vi "Picolog Get Unit Info.vi"(8 "Error In":errorcluster, 11 "Instrument Handle In":i16=1) -> (0 "Error Out":errorcluster, 1 "Unit Info":string, 3 "Instrument Handle Out":i16)   [LabVIEW 2016]
uses:
  usbtc08.dll
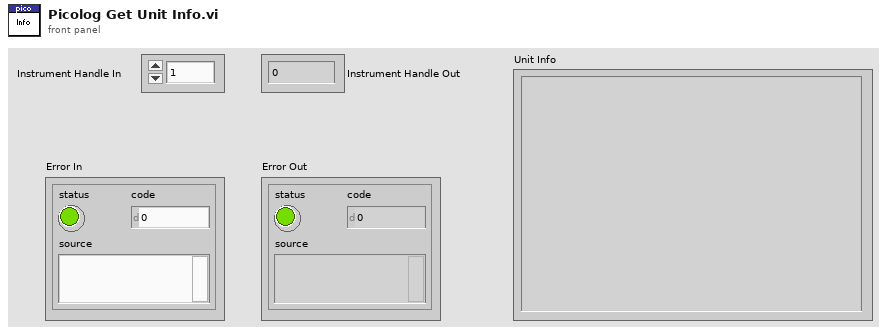
[diagram p1: front panel]
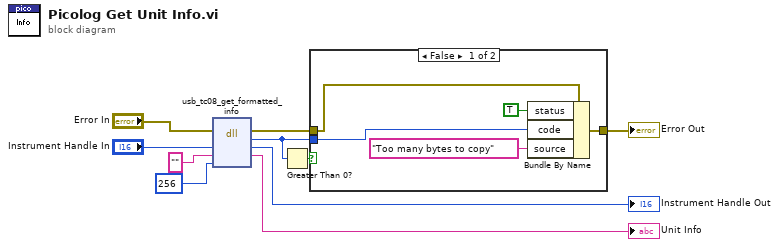
[diagram p0: block diagram]
diagram:
  n1 = dll-call lib="usbtc08.dll" fn="usb_tc08_get_formatted_info"(error in="Error In", "handle"="Instrument Handle In", "info"="", "string_length"=i16 256 ("String Length")) -> (error out=w7:errorcluster, "return type"=w3:i16, "handle"=→"Instrument Handle Out":i16, "info"=→"Unit Info":string)  [unwired: 3 in, 1 out]
  n2 = Greater Than 0?(x=w3) -> (x > 0?=w8:bool)
  n3 = case shown="False" w8 {
    tunnel: w7 -> [w15 w16]
    tunnel: [w14 w16] -> w6
    tunnel: w3 -> [w11 _]
    frame False {
      n4 = Bundle By Name(cluster=w15, "status"=TRUE, "code"=w11, "source"="Too many bytes to copy") -> (w14:errorcluster)
    }
    frame True {
    }
  }
  "Error Out" <- w6
